vi "XX-I16.vi"(8 "单位":dbl=16960.0, 9 "下限":i16=-90, 10 "上限":i16=90, 11 "数值输入":i16) -> (3 "输出":i16)   [LabVIEW 2012]
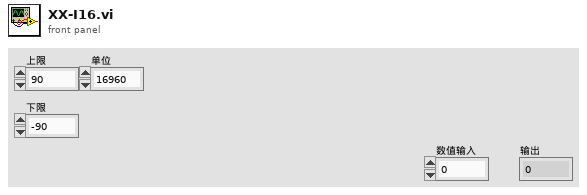
[diagram p1: front panel]
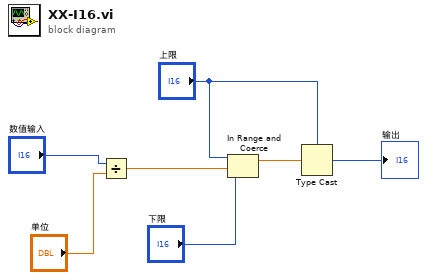
[diagram p0: block diagram]
diagram:
  n1 = Divide(x="数值输入", y="单位") -> (x/y=w3:dbl)
  n2 = In Range and Coerce(upper limit="上限", x=w3, lower limit="下限") -> (coerced(x)=w4:dbl)  [unwired: 1 out]
  n3 = Type Cast(type="上限", x=w4) -> (*(type *) &x=→"输出":i16)
